vi "spot size 2D.vi"(6 "half width for 2nd mom cut":sgl, 7 "Threshold for 2nd mom":dbl=0.05 format="%#_13g", 8 "error in (no error)":errorcluster, 9 "X Centroid":sgl, 10 "Y Centroid":sgl, 11 "Refnum in":T1) -> (0 "w0y via 2nd mom":sgl, 1 "w0x via 2nd mom":sgl, 2 "FWHMx (pix)":dbl, 3 "FWHMy (pix)":dbl, 4 "error out":errorcluster)   [LabVIEW 2020]
uses:
  IMAQ Image.ctl
  NI_Vision_Development_Module.lvlib
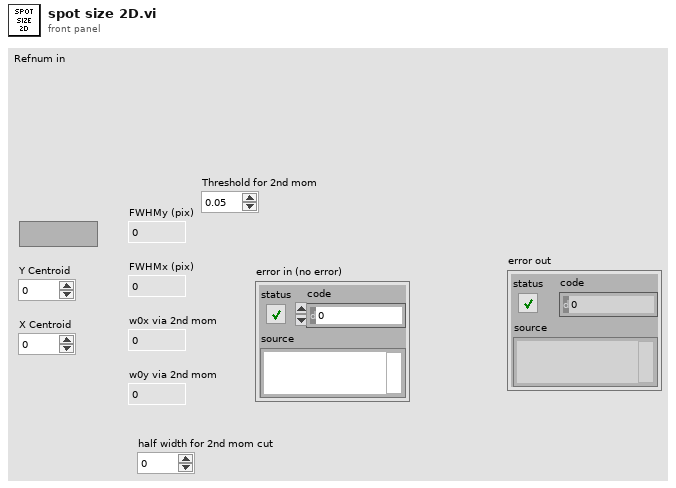
[diagram p1: front panel]
types:
  T1 = typedef "IMAQ Image.ctl" = refnum<image>
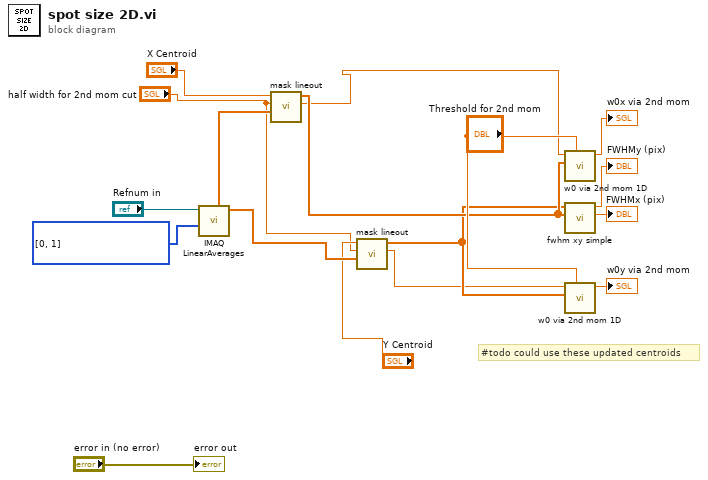
[diagram p0: block diagram]
diagram:
  w13 = i32[] [0, 1] items=["X Axis Averages", "Y Axis Averages", "X + Y Axis Averages", "X - Y Axis Averages"] ("Averages")
  # "#todo could use these updated centroids"
  n1 = call "IMAQ LinearAverages"("Averages"=w13, "Image Src"="Refnum in") -> ("Y Axis Averages"=w6:sgl[], "X Axis Averages"=w9:sgl[])  [unwired: 2 in, 6 out]
  n2 = call "mask lineout.vi"("X Axis Averages"=w9, "half width for 2nd mom cut"="half width for 2nd mom cut", "X Centroid"="X Centroid") -> ("updated centroid"=w2:dbl, "Waveform Graph"=w8:dbl[])  [unwired: 7 in]
  n3 = call "mask lineout.vi"("X Axis Averages"=w6, "half width for 2nd mom cut"="half width for 2nd mom cut", "X Centroid"="Y Centroid") -> ("updated centroid"=w1:dbl, "Waveform Graph"=w7:dbl[])  [unwired: 7 in]
  n4 = call "w0 via 2nd mom 1D.vi"("Threshold for 2nd mom"="Threshold for 2nd mom", "Input array"=w8, "Centroid"=w2) -> ("w0 via 2nd mom"=→"w0x via 2nd mom":sgl)  [unwired: 8 in]
  n5 = call "fwhm xy simple.vi"("X Axis Averages"=w8, "Y Axis Averages"=w7) -> ("FWHM (pix) 2"=→"FWHMx (pix)":dbl, "FWHM (pix)"=→"FWHMy (pix)":dbl)  [unwired: 8 in]
  n6 = call "w0 via 2nd mom 1D.vi"("Threshold for 2nd mom"="Threshold for 2nd mom", "Input array"=w7, "Centroid"=w1) -> ("w0 via 2nd mom"=→"w0y via 2nd mom":sgl)  [unwired: 8 in]
  "error out" <- "error in (no error)"
